vi "Cleanup Session.vi"(8 "error in":errorcluster, 11 "Plugin in":refnum<class "Configure Visa Device Channels.lvclass">) -> (0 "error out":errorcluster, 3 "Plugin out":refnum<class "Configure Visa Device Channels.lvclass">)   [LabVIEW 2026, in "Configure Visa Device Channels.lvlib" / "Configure Visa Device Channels.lvclass"]
uses:
  Configure Visa Device Channels.lvclass
  Configure Visa Device Channels.lvclass/Configure Visa Device Channels.ctl
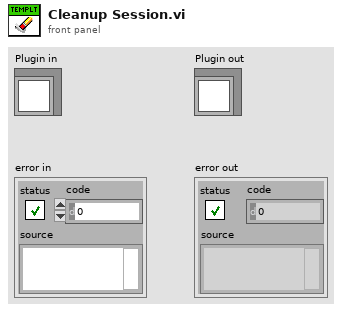
[diagram p1: front panel]
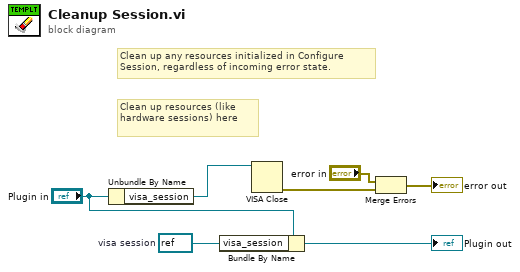
[diagram p0: block diagram]
diagram:
  w7 = refnum<visa-resource-name> refnum  # visa session
  # "Clean up resources (like hardware sessions) here"
  # "Clean up any resources initialized in Configure Session, regardless of incoming error state."
  n1 = Unbundle By Name("Plugin in") -> ("visa_session"=w4:refnum<visa-resource-name>)
  n2 = Bundle By Name(cluster="Plugin in", "visa_session"=w7) -> (→"Plugin out":refnum<class "Configure Visa Device Channels.lvclass">)
  n3 = VISA Close(VISA resource name=w4) -> (error out=w2:errorcluster)  [unwired: 1 in]
  n4 = Merge Errors("error in", w2) -> (→"error out":errorcluster)
